vi "Unflatten.vi"(8 "Error In":errorcluster, 10 "Type/Default":variant, 11 "Response in":refnum<class "Request.lvclass">) -> (0 "Error Out":errorcluster, 2 "Value":variant, 3 "Response out":refnum<class "Request.lvclass">)   [LabVIEW 2023, in "Request.lvclass"]
doc: "Helper VI that attempts to unflatten the Request Body as the specified data type. Primarily used in conjunction with Control Referenece/Event Handler Endpoints."
uses:
  Request.lvclass
  Request.lvclass/Request.ctl
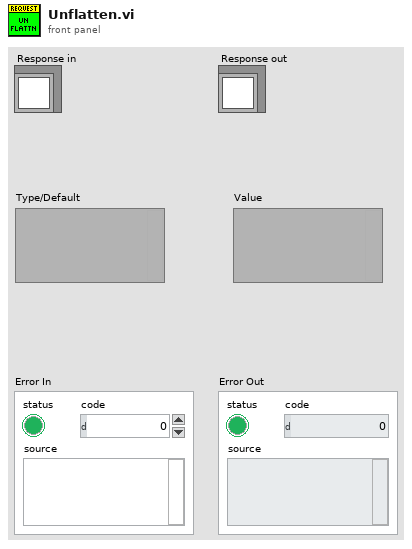
[diagram p1: front panel]
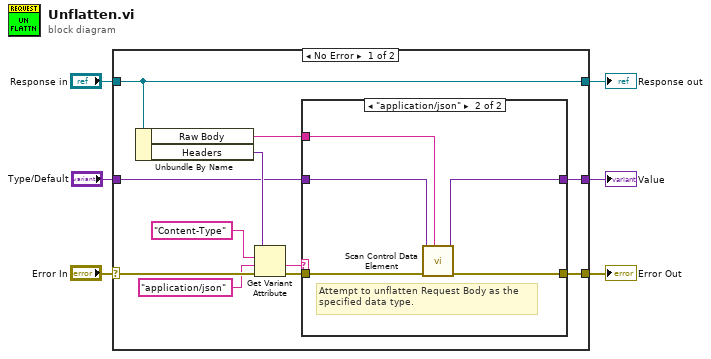
[diagram p0: block diagram]
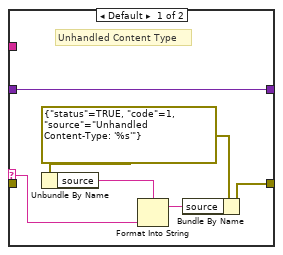
[diagram p2: hidden frame]
diagram:
  n1 = case shown="No Error" "Error In" {
    selector: "Error In" -> [w17 w31]
    tunnel: [w10 w31] -> w5
    tunnel: [w16 w30] -> w3
    tunnel: "Response in" -> [w16 w30]
    tunnel: [w9 w29] -> w2
    tunnel: "Type/Default" -> [w8 w29]
    frame No Error {
      n2 = Unbundle By Name(w16) -> ("Raw Body"=w7:string, "Headers"=w15:variant)
      n3 = Get Variant Attribute(Variant=w15, name="Content-Type", default value (empty Variant)="application/json" ("name"), error in=w17) -> (value=w11:string, error out=w12:errorcluster)  [unwired: 2 out]
      n4 = case shown="\"application/json\"" w11 {
        selector: w11 -> [w19 _]
        tunnel: w12 -> [_ w28]
        tunnel: [w22 w27] -> w10
        tunnel: [w23 w26] -> w9
        tunnel: w8 -> [w23 w24]
        tunnel: w7 -> [_ w25]
        frame Default {
          w18 = errorcluster {"status"=TRUE, "code"=1, "source"="Unhandled Content-Type: '%s'"} ("error out")
          # "Unhandled Content Type"
          n5 = Unbundle By Name(w18) -> ("source"=w20:string)
          n6 = Format Into String(format string=w20, w19) -> (resulting string=w21:string)  [unwired: 2 in, 1 out]
          n7 = Bundle By Name(cluster=w18, "source"=w21) -> (w22:errorcluster)
        }
        frame "application/json" {
          # "Attempt to unflatten Request Body as the\nspecified data type."
          n8 = call "Scan Control Data Element.vi"("Body"=w25, "error in (no error)"=w28, "Type/Default in"=w24) -> ("error out"=w27:errorcluster, "Type/Default out"=w26:variant)  [unwired: 7 in]
        }
      }
    }
    frame Error {
    }
  }
  "Error Out" <- w5
  "Response out" <- w3
  "Value" <- w2
